vi "Config File Read.vi"(6 "Controls Excluded":refnum<vi>[](array[refnum]), 8 "Error In":errorcluster, 10 "Path":path, 11 "Controls In":refnum<vi>[](array[refnum])) -> (0 "Error Out":errorcluster, 1 "Fixe Exists?":bool, 2 "Values":variant[](array[variant]), 3 "Controls Out":refnum<vi>[](array[refnum]))   [LabVIEW 2015]
uses:
  <vilib>/Utility/config.llb/Read Key (String).vi
  <vilib>/Utility/config.llb/NI_LVConfig.lvlib
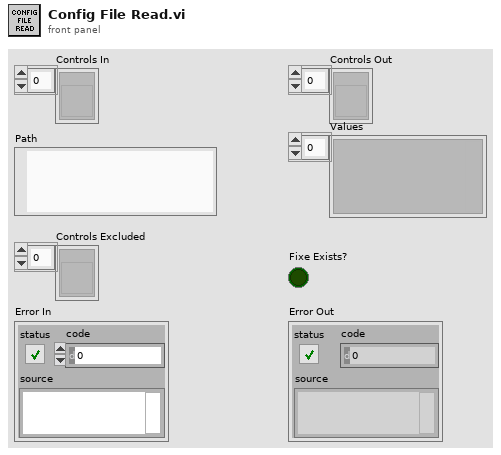
[diagram p1: front panel]
types:
  T1 = typedef "NI_LVConfig.lvlib/Config Data RefNum.ctl" = refnum<k1>
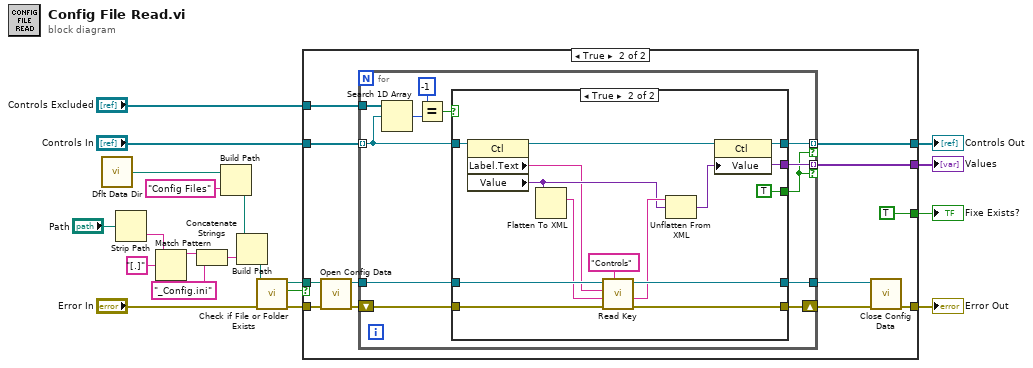
[diagram p0: block diagram]
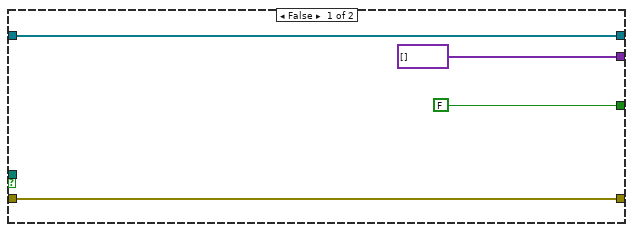
[diagram p2: hidden frame]
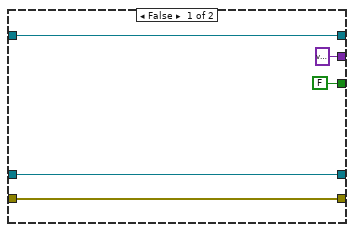
[diagram p3: hidden frame]
diagram:
  n1 = call <vilib>:"Dflt Data Dir.vi"() -> ("App:Default Data Directory"=w3:path)
  n2 = Strip Path(path="Path") -> (name=w20:string)  [unwired: 1 out]
  n3 = Match Pattern(string=w20, regular expression="[.]" ("search string")) -> (before substring=w18:string)  [unwired: 1 in, 3 out]
  n4 = Concatenate Strings(w18, "_Config.ini") -> (w16:string)
  n5 = Build Path(base path=w3, name or relative path="Config Files") -> (appended path=w1:path)
  n6 = Build Path(base path=w1, name or relative path=w16) -> (appended path=w10:path)
  n7 = call <vilib>:"Check if File or Folder Exists.vi"("error in (no error)"="Error In", "path"=w10) -> ("error out"=w11:errorcluster, "file or folder exists?"=w6:bool, "dup path"=w9:path)  [unwired: 7 in]
  n8 = case shown="True" w6 {
    tunnel: "Controls In" -> [w24 w32]
    tunnel: [w21 w31] -> w13
    tunnel: w11 -> [w21 w30]
    tunnel: w9 -> [_ w29]
    tunnel: [w24 w28] -> w8
    tunnel: [variant[] [] w27] -> w7
    tunnel: [FALSE TRUE] -> w5
    tunnel: "Controls Excluded" -> [_ w25]
    frame False {
    }
    frame True {
      n9 = call <vilib>:"Open Config Data.vi"("error in (no error)"=w30, "configuration file path"=w29) -> ("error out"=w35:errorcluster, "refnum"=w36:T1)  [unwired: 1 in, 7 out]
      n10 = for {
        shift-right: [w46] -> w34
        shift-left: w35 -> [w47]
        tunnel: w32 -> [w39] mode=indexing
        tunnel: [w44] -> w27 mode=indexing if=w37
        tunnel: [w43] -> w28 mode=indexing if=w37
        tunnel: w25 -> [w42]
        tunnel: w36 -> [w48]
        tunnel: [w45] -> w33
        n11 = Search 1D Array(1D array=w42, element=w39) -> (index of element=w41:i32)  [unwired: 1 in]
        n12 = Equal?(x=-1, y=w41) -> (x = y?=w38:bool)
        n13 = case shown="True" w38 {
          tunnel: w48 -> [w50 w67]
          tunnel: w47 -> [w49 w66]
          tunnel: [w49 w64] -> w46
          tunnel: [w50 w63] -> w45
          tunnel: [variant ("Value") w58] -> w44
          tunnel: [w53 w57] -> w43
          tunnel: w39 -> [w53 w55]
          tunnel: [FALSE TRUE] -> w37
          frame False {
          }
          frame True {
            n14 = property class="Ctl"(reference=w55) -> (reference out=w56:refnum<vi>, "Label.Text"=w59:string, "Value"=w60:variant)  [unwired: 1 in, 1 out]
            n15 = Flatten To XML(anything=w60) -> (xml string=w62:string)
            n16 = call-poly <vilib>:"Read Key.vi"("section"="Controls", "error in (no error)"=w66, "default value"=w62, "key"=w59, "refnum"=w67) -> ("error out"=w64:errorcluster, "value"=w61:string, "refnum out"=w63:T1)  [unwired: 3 in, 1 out]
            n17 = Unflatten From XML(xml string=w61, type=w60) -> (value=w58:variant)  [unwired: 1 in, 1 out]
            n18 = property class="Ctl"(reference=w56, "Value"=w58) -> (reference out=w57:refnum<vi>)  [unwired: 1 in, 1 out]
          }
        }
      }
      n19 = call <vilib>:"Close Config Data.vi"("error in (no error)"=w34, "refnum"=w33) -> ("error out"=w31:errorcluster)  [unwired: 1 in, 8 out]
    }
  }
  "Error Out" <- w13
  "Controls Out" <- w8
  "Values" <- w7
  "Fixe Exists?" <- w5
